vi "Main_FPGA old.vi"() -> ()   [LabVIEW 2018]
uses:
  <vilib>/rvi/eio/common/nirviEmuTemplateMethod_errors.vi
  <vilib>/rvi/Emulation/niFpgaGetClockAttributes.vi
  <vilib>/rvi/Emulation/niFpgaSctlEmulationGetInTimedLoop.vi
  <vilib>/rvi/Emulation/niFpgaEmulationReportErrorSimple.vi
  <vilib>/rvi/Emulation/niFpgaProcessEmulError.vi
  <vilib>/rvi/Emulation/niFpgaCriticalErrorInLSC.vi
  <vilib>/eio/EIONode/EIONode.xnode
  <vilib>/addons/control/pid/fpga.llb/XNode/niFpgaPID.xnode
panel:
  out "Mod6/unitR":bool
  out "Mod6/unitL":bool
  in  "Speed Loop Rate":u32=1000
  out "Mod8/AI15":fxp<+/-,24,5>
  out "Mod8/AI5":fxp<+/-,24,5>
  out "Mod8/AI4":fxp<+/-,24,5>
  out "Speed_cmd":fxp<+/-,17,6>
  in  "FeedFw_Ena":bool
  in  "ACC_FeedFw":fxp<+/-,16,5>
  out "Acc_2":fxp<+/-,36,10>
  out "Acc_1":fxp<+/-,36,10>
  in  "E-Acc_2":T1={"Gain"=1.0, "OffSet"=0.0}
  in  "E-Acc_1":T1={"Gain"=1.0, "OffSet"=0.0}
  in  "Speed Control Soll (%)":fxp<+/-,16,5>
  in  "Parameter Speed Control":fxp<+/-,16,5>
  in  "PID gains":T2={"proportional gain (Kc)"=1.5, "integral gain (Kc*Ts/Ti)"=0.19921875, "derivative gain (Kc*Td/Ts)"=0.0}
  in  "output range":T3={"output high"=10.0, "output low"=0.0}
  in  "Regler Speed Control":bool
  in  "Ist Speed Control":fxp<+/-,16,5>
  in  "Count (mSec) Fahrhebel":u32=25
  out "Tick Count(mSec) Hydraulic Wave":u32
  out "Count Hydraulic  Wave":i64
  out "Mod6/Fuel Transmitter":bool
  out "Mod6/DI30":bool
  out "Tick Count(mSec) Hydraulic":u32
  out "Count Hydraulic":i64
  in  "Mod7/Hydraulic clutch Set point":fxp<+/-,20,5>
  in  "Mod7/Hydraulic pump actuator Soll":fxp<+/-,20,5>
  in  "Mod7/Out 2":fxp<+/-,20,5>
  in  "Mod7/Out 1":fxp<+/-,20,5>
  out "DM Count":i64
  out "Tick Count(mSec)":u32
  in  "Mod4/DO30":bool
  in  "Mod4/Release Brake M":bool
  in  "Mod4/Richtung Engine Speed M":bool
  in  "Mod4/Release Engine Speed M":bool
  in  "Mod4/Richtung Up M":bool
  in  "Mod4/Release Up M":bool
  out "Mod6/End Position DOWN M":bool
  out "Mod6/DOWN M":bool
  out "Mod6/UP M":bool
  out "Mod6/End Position UP M":bool
  in  "Mod7/Up M Set point":fxp<+/-,20,5>
  in  "Mod7/Torque M Set point":fxp<+/-,20,5>
  out "Mod8/Engine Speed M":fxp<+/-,24,5>
  out "Mod8/Up M":fxp<+/-,24,5>
  in  "Mod4/Clutch":bool
  in  "Mod4/Temperature Control Release":bool
  in  "Mod4/Temperature Control OFF":bool
  in  "Mod4/Calibration ON Brake H":bool
  in  "Mod4/Unit ON Brake H":bool
  in  "Mod4/Brake Performance ON Brake H":bool
  in  "Mod4/Oil ON":bool
  in  "Mod3/Calibration Brake R":bool
  in  "Mod3/Unit ON Brake R":bool
  in  "Mod3/Brake Performance ON Brake R":bool
  in  "Mod3/Horn":bool
  in  "Mod3/DO20":bool
  in  "Mod3/Speed Control Release":bool
  in  "Mod3/DO18":bool
  in  "Mod3/Flashing light":bool
  in  "Mod3/Calibration ON Brake L":bool
  in  "Mod3/Unit ON Brake L":bool
  in  "Mod3/Brake Performance ON Brake L":bool
  in  "Mod3/Converter Clutch ON":bool
  in  "Mod3/Fuel Pump ON":bool
  in  "Mod3/Engine Ignition ON":bool
  in  "Mod3/Start Engine":bool
  in  "Mod3/Engine Pre Glow ON":bool
  in  "Cooling  Set point (°C)":fxp<+/-,16,5>
  in  "Heater Set point (°C)":fxp<+/-,16,5>
  in  "Alarm 24 ON":bool
  in  "Alarm 23 ON":bool
  in  "Alarm 22 ON":bool
  in  "Alarm 21 ON":bool
  in  "Alarm 20 ON":bool
  in  "Alarm 19 ON":bool
  in  "Alarm 18 ON":bool
  in  "Alarm 17 ON":bool
  in  "Alarm 16 ON":bool
  in  "Alarm 15 ON":bool
  in  "Alarm 14 ON":bool
  in  "Alarm 13 ON":bool
  in  "Alarm 12 ON":bool
  in  "Alarm 11 ON":bool
  in  "Alarm 10 ON":bool
  in  "Alarm 9 ON":bool
  in  "Alarm 8 ON":bool
  in  "Alarm 7 ON":bool
  in  "Alarm 6 ON":bool
  in  "Alarm 5 ON":bool
  in  "Alarm 4 ON":bool
  in  "Alarm 3 ON":bool
  out "Alarm":bool
  in  "Alarm 2 ON":bool
  in  "Alarm 1 ON":bool
  in  "Alarm ON":bool
  in  "STOP":bool
  out "Mod8/Kal 2 Brake H":fxp<+/-,24,5>
  out "Mod8/Kal 1 Brake H":fxp<+/-,24,5>
  out "Mod8/Kal 2 Brake R":fxp<+/-,24,5>
  out "Mod8/Kal 1 Brake R":fxp<+/-,24,5>
  out "Mod8/Kal 2 Brake L":fxp<+/-,24,5>
  out "Mod8/Kal 1 Brake L":fxp<+/-,24,5>
  out "Mod8/Engine Speed Wave Sensor":fxp<+/-,24,5>
  out "Mod8/Speed Control":fxp<+/-,24,5>
  in  "Mod3/System Reset/ON":bool
  out "Mod6/Clutch open":bool
  out "Mod6/Clutch closed":bool
  out "Mod6/Alarm 25 Basement":bool
  out "Mod6/Unit L-R":bool
  out "Mod6/Unit H":bool
  out "Mod6/Unit H-L-R":bool
  out "Mod6/Sytem Ready":bool
  out "Mod6/Watchdog Ready":bool
  out "Mod6/Alarm 2 Brake back":bool
  out "Mod6/Alarm 1 Brake back":bool
  out "Mod6/Temperature Brake back":bool
  out "Mod6/Ready Brake back":bool
  out "Mod6/Error Brake back":bool
  out "Mod6/Alarm 24 Overload Warning Oil Heating":bool
  out "Mod6/Alarm 23 Overload Warning Oil Pump":bool
  out "Mod6/Alarm 22 max Oil Pressure":bool
  out "Mod6/Alarm 21 min Oil Pressure":bool
  out "Mod6/Alarm 20 max Oil Temperature":bool
  out "Mod6/Alarm 18 Oil Level":bool
  out "Mod6/Alarm 19 min Oil Pressure":bool
  out "Mod6/Alarm 17 Oil Pressure Difference":bool
  out "Mod5/Alarm 2 Brake R":bool
  out "Mod5/Alarm 1 Brake R":bool
  out "Mod5/Temperature Brake R":bool
  out "Mod5/Ready Brake R":bool
  out "Mod5/Error Brake R":bool
  out "Mod5/Alarm 16 Fundament 4":bool
  out "Mod5/Alarm 15 Fundament 3":bool
  out "Mod5/Alarm 14 Fundament 2":bool
  out "Mod5/Alarm 13 Fundament 1":bool
  out "Mod5/Alarm 12 Spring Element":bool
  out "Mod5/Alarm 11 Watchdog":bool
  out "Mod5/Alarm 10 Fuel Depot":bool
  out "Mod5/Alarm 9 IGBT_ON":bool
  out "Mod5/Alarm 2 Brake L":bool
  out "Mod5/Alarm 1 Brake L":bool
  out "Mod5/Temperature Brake L":bool
  out "Mod5/Ready Brake L":bool
  out "Mod5/Error Brake L":bool
  out "Mod5/Alarm 8 Cooling Water":bool
  out "Mod5/Alarm 7 Exhaust":bool
  out "Mod5/Alarm 6 CO2":bool
  out "Mod5/Alarm 5 Clutch":bool
  out "Mod5/Alarm 4 Speed Control":bool
  out "Mod5/Alarm 3 Flow Control Unit":bool
  out "Mod5/Alarm 2 Gas":bool
  out "Mod5/Alarm 1 Fire":bool
  out "Mod2/Engine Speed  H":fxp<+/-,20,5>
  out "Mod2/Engine Speed R":fxp<+/-,20,5>
  out "Mod2/Engine Speed  L":fxp<+/-,20,5>
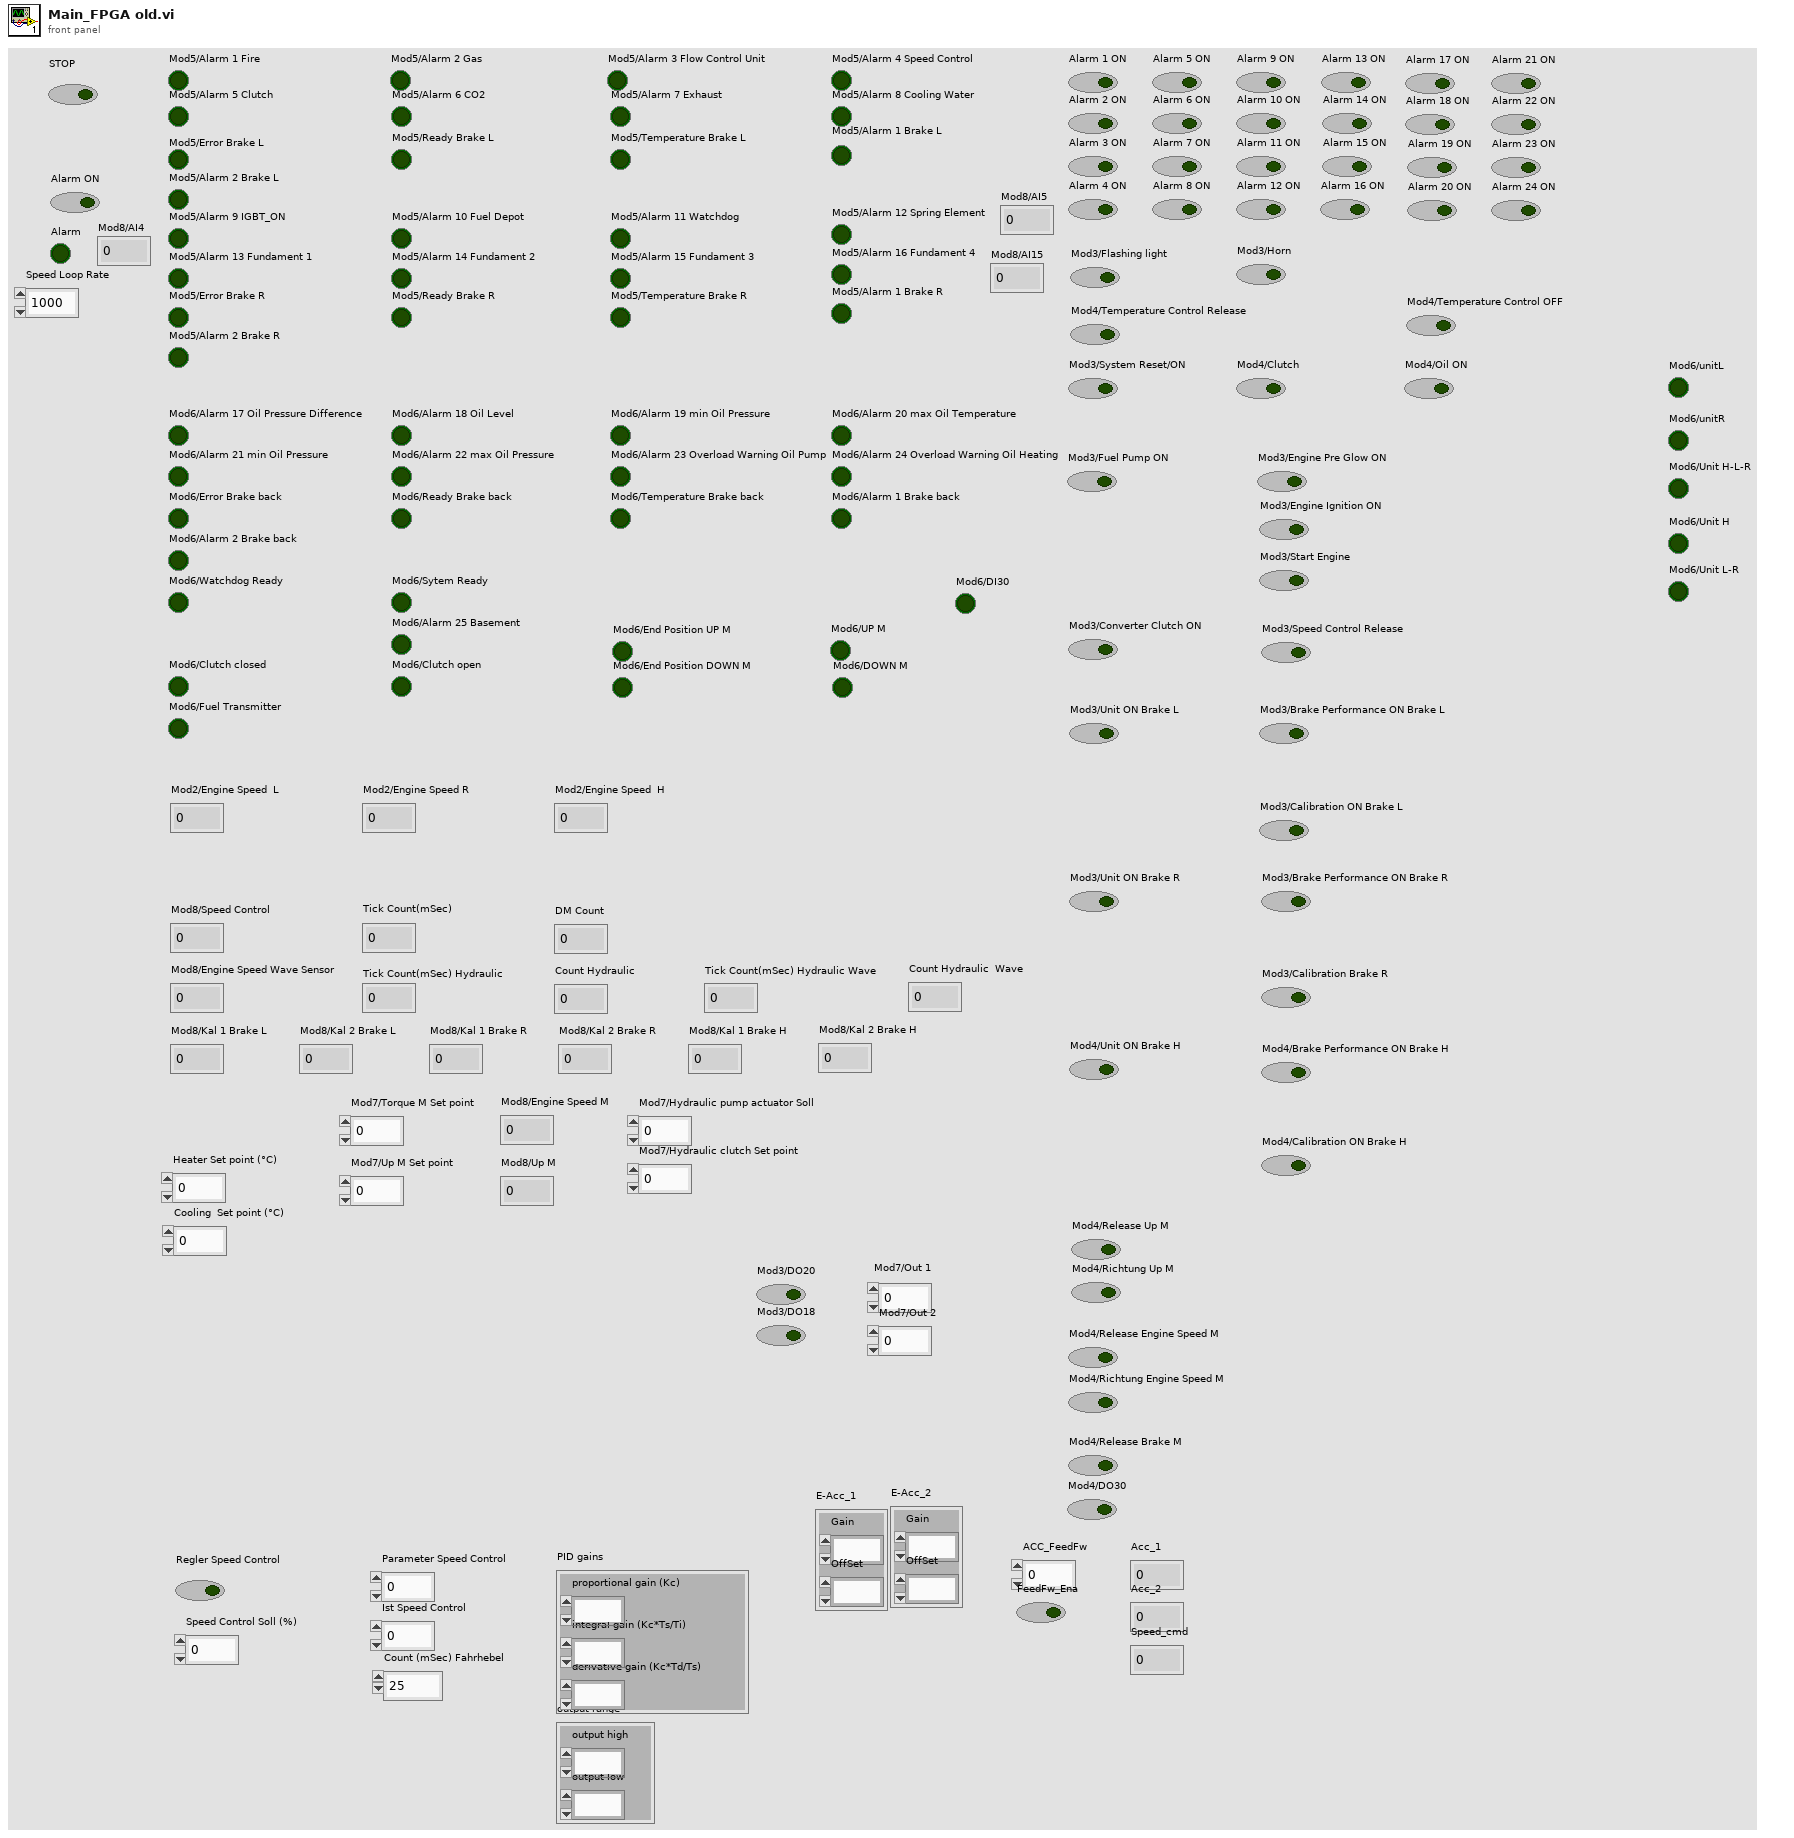
[diagram p1: front panel]
types:
  T1 = cluster{"Gain":fxp<+/-,20,5>, "OffSet":fxp<+/-,20,5>}
  T2 = cluster{"proportional gain (Kc)":fxp<+/-,16,8>, "integral gain (Kc*Ts/Ti)":fxp<+/-,16,8>, "derivative gain (Kc*Td/Ts)":fxp<+/-,16,8>}
  T3 = cluster{"output high":fxp<+/-,16,5>, "output low":fxp<+/-,16,5>}
  T4 = cluster{"proportional gain (Kc)":i16, "integral gain (Kc*Ts/Ti)":i16, "derivative gain (Kc*Td/Ts)":i16}
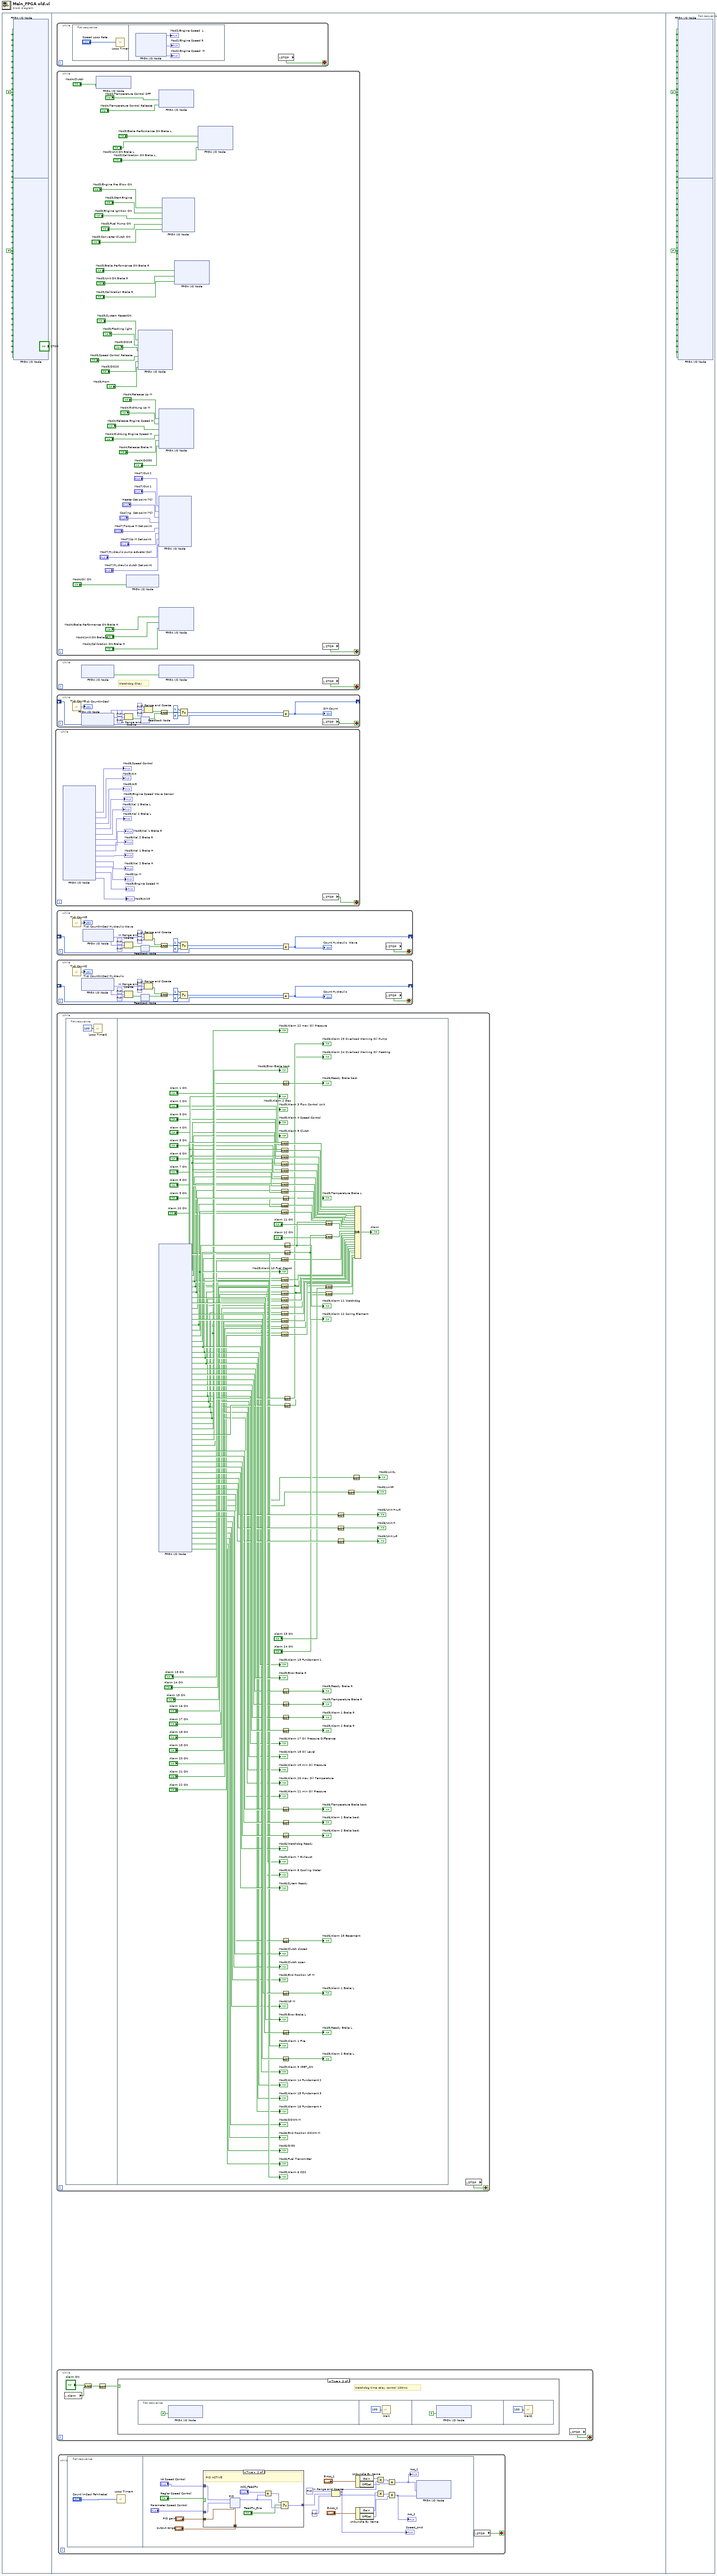
[diagram p0: block diagram]
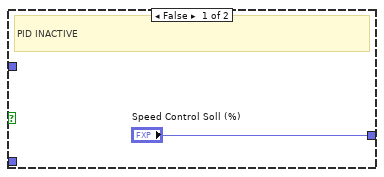
[diagram p2: hidden frame]
diagram:
  n1 = flat-sequence {
    frame #0 {
      w1 = FALSE ("Mod4/DO0")
      w2 = FALSE ("Mod3/DO0")
      n2 = xnode "FPGA I/O Node"("Mod4/DO0"=w1, "Mod4/DO1"=w1, "Mod4/DO2"=w1, "Mod4/DO3"=w1, "Mod4/DO4"=w1, "Mod4/DO5"=w1, "Mod4/DO6"=w1, "Mod4/DO7"=w1, "Mod4/DO8"=w1, "Mod4/DO9"=w1, "Mod4/DO10"=w1, "Mod4/DO11"=w1, "Mod4/DO12"=w1, "Mod4/DO13"=w1, "Mod4/DO14"=w1, "Mod4/DO15"=w1, "Mod4/DO16"=w1, "Mod4/DO17"=w1, "Mod4/DO18"=w1, "Mod4/DO19"=w1, "Mod4/DO20"=w1, "Mod4/DO21"=w1, "Mod4/DO22"=w1, "Mod4/DO23"=w1, "Mod4/DO24"=w1, "Mod4/DO25"=w1, "Mod4/DO26"=w1, "Mod4/DO27"=w1, "Mod4/DO28"=w1, "Mod4/DO29"=w1, "Mod4/DO30"=w1, "Mod4/DO31"=w1) -> ()  [unwired: 32 in, 32 out]
      n3 = xnode "FPGA I/O Node"("Mod3/DO0"=w2, "Mod3/DO1"=w2, "Mod3/DO2"=w2, "Mod3/DO3"=w2, "Mod3/DO4"=w2, "Mod3/DO5"=w2, "Mod3/DO6"=w2, "Mod3/DO7"=w2, "Mod3/DO8"=w2, "Mod3/DO9"=w2, "Mod3/DO10"=w2, "Mod3/DO11"=w2, "Mod3/DO12"=w2, "Mod3/DO13"=w2, "Mod3/DO14"=w2, "Mod3/DO15"=w2, "Mod3/DO16"=w2, "Mod3/DO17"=w2, "Mod3/DO18"=w2, "Mod3/DO19"=w2, "Mod3/DO20"=w2, "Mod3/DO21"=w2, "Mod3/DO22"=w2, "Mod3/DO23"=w2, "Mod3/DO24"=w2, "Mod3/DO25"=w2, "Mod3/DO26"=w2, "Mod3/DO27"=w2, "Mod3/DO28"=w2, "Mod3/DO29"=w2, "Mod3/DO30"=w2, "Mod3/DO31"=w2) -> ()  [unwired: 32 in, 32 out]
    }
    frame #1 {
      n4 = while {
        stop <- w6 stop-if-true
        n5 = xnode "FPGA I/O Node"() -> ("Mod8/AI3"=→"Mod8/Speed Control":fxp<+/-,24,5>, "Mod8/AI4"=→"Mod8/AI4":fxp<+/-,24,5>, "Mod8/AI5"=→"Mod8/AI5":fxp<+/-,24,5>, "Mod8/AI6"=→"Mod8/Engine Speed Wave Sensor":fxp<+/-,24,5>, "Mod8/AI7"=→"Mod8/Kal 1 Brake L":fxp<+/-,24,5>, "Mod8/AI8"=→"Mod8/Kal 2 Brake L":fxp<+/-,24,5>, "Mod8/AI9"=→"Mod8/Kal 1 Brake R":fxp<+/-,24,5>, "Mod8/AI10"=→"Mod8/Kal 2 Brake R":fxp<+/-,24,5>, "Mod8/AI11"=→"Mod8/Kal 1 Brake H":fxp<+/-,24,5>, "Mod8/AI12"=→"Mod8/Kal 2 Brake H":fxp<+/-,24,5>, "Mod8/AI13"=→"Mod8/Up M":fxp<+/-,24,5>, "Mod8/AI14"=→"Mod8/Engine Speed M":fxp<+/-,24,5>, "Mod8/AI15"=→"Mod8/AI15":fxp<+/-,24,5>)  [unwired: 16 in, 19 out]
        n6 = local read "STOP"() -> (w6:bool)
      }
      n7 = while {
        stop <- w17 stop-if-true
        n8 = flat-sequence {
          frame #0 {
            n9 = call "Loop Timer"("Count(uSec)"="Speed Loop Rate") -> ()  [unwired: 1 out]
          }
          frame #1 {
            n10 = xnode "FPGA I/O Node"() -> ("Mod2/AI0"=→"Mod2/Engine Speed  L":fxp<+/-,20,5>, "Mod2/AI1"=→"Mod2/Engine Speed R":fxp<+/-,20,5>, "Mod2/AI2"=→"Mod2/Engine Speed  H":fxp<+/-,20,5>)  [unwired: 3 in, 3 out]
          }
        }
        n11 = local read "STOP"() -> (w17:bool)
      }
      n12 = while {
        stop <- w167 stop-if-true
        n13 = xnode "FPGA I/O Node"("Mod4/DO24"="Mod4/Clutch") -> ()  [unwired: 1 in, 1 out]
        n14 = xnode "FPGA I/O Node"("Mod4/DO5"="Mod4/Oil ON") -> ()  [unwired: 1 in, 1 out]
        n15 = xnode "FPGA I/O Node"("Mod3/DO16"="Mod3/System Reset/ON", "Mod3/DO17"="Mod3/Flashing light", "Mod3/DO18"="Mod3/DO18", "Mod3/DO19"="Mod3/Speed Control Release", "Mod3/DO20"="Mod3/DO20", "Mod3/DO21"="Mod3/Horn") -> ()  [unwired: 6 in, 6 out]
        n16 = xnode "FPGA I/O Node"("Mod4/DO18"="Mod4/Temperature Control OFF", "Mod4/DO19"="Mod4/Temperature Control Release") -> ()  [unwired: 2 in, 2 out]
        n17 = xnode "FPGA I/O Node"("Mod4/DO25"="Mod4/Release Up M", "Mod4/DO26"="Mod4/Richtung Up M", "Mod4/DO27"="Mod4/Release Engine Speed M", "Mod4/DO28"="Mod4/Richtung Engine Speed M", "Mod4/DO29"="Mod4/Release Brake M", "Mod4/DO30"="Mod4/DO30") -> ()  [unwired: 6 in, 6 out]
        n18 = xnode "FPGA I/O Node"("Mod7/AO2"="Mod7/Out 2", "Mod7/AO1"="Mod7/Out 1", "Mod7/AO3"="Heater Set point (°C)", "Mod7/AO4"="Cooling  Set point (°C)", "Mod7/AO5"="Mod7/Torque M Set point", "Mod7/AO6"="Mod7/Up M Set point", "Mod7/AO7"="Mod7/Hydraulic pump actuator Soll", "Mod7/AO8"="Mod7/Hydraulic clutch Set point") -> ()  [unwired: 8 in, 8 out]
        n19 = xnode "FPGA I/O Node"("Mod4/DO10"="Mod4/Brake Performance ON Brake H", "Mod4/DO11"="Mod4/Unit ON Brake H", "Mod4/DO12"="Mod4/Calibration ON Brake H") -> ()  [unwired: 3 in, 3 out]
        n20 = xnode "FPGA I/O Node"("Mod3/DO0"="Mod3/Engine Pre Glow ON", "Mod3/DO1"="Mod3/Start Engine", "Mod3/DO2"="Mod3/Engine Ignition ON", "Mod3/DO3"="Mod3/Fuel Pump ON", "Mod3/DO4"="Mod3/Converter Clutch ON") -> ()  [unwired: 5 in, 5 out]
        n21 = xnode "FPGA I/O Node"("Mod3/DO26"="Mod3/Brake Performance ON Brake R", "Mod3/DO27"="Mod3/Unit ON Brake R", "Mod3/DO28"="Mod3/Calibration Brake R") -> ()  [unwired: 3 in, 3 out]
        n22 = xnode "FPGA I/O Node"("Mod3/DO10"="Mod3/Brake Performance ON Brake L", "Mod3/DO11"="Mod3/Unit ON Brake L", "Mod3/DO12"="Mod3/Calibration ON Brake L") -> ()  [unwired: 3 in, 3 out]
        n23 = local read "STOP"() -> (w167:bool)
      }
      n24 = while {
        stop <- w177 stop-if-true
        # "Watchdog Okay"
        n25 = xnode "FPGA I/O Node"() -> ("Mod6/DI16"=w178:bool)  [unwired: 1 in, 1 out]
        n26 = xnode "FPGA I/O Node"("Mod4/DO17"=w178) -> ()  [unwired: 1 in, 1 out]
        n27 = local read "STOP"() -> (w177:bool)
      }
      n28 = while {
        shift-right: [w121] -> _
        shift-left: _ -> [w122]
        stop <- w119 stop-if-true
        n29 = call "Tick Count"() -> ("Tick Count(mSec)"=→"Tick Count(mSec)":u32)
        n30 = xnode "FPGA I/O Node"() -> ("Mod8/AI14"=w116:fxp<+/-,24,5>)  [unwired: 1 in, 1 out]
        n31 = In Range and Coerce(upper limit=fxp<+/-,24,5> 3.0, x=w116, lower limit=fxp<+/-,24,5> 0.0) -> (In Range?=w117:bool)  [unwired: 1 out]
        n32 = feedback-in #1(w117) -> ()
        n33 = feedback #1() -> (w118:bool)  [unwired: 1 in]
        n34 = In Range and Coerce(upper limit=fxp<+/-,24,5> 6.0, x=w116, lower limit=fxp<+/-,24,5> 3.0) -> (In Range?=w113:bool)  [unwired: 1 out]
        n35 = And(x=w113, y=w118) -> (x .and. y?=w126:bool)
        n36 = Select(t=i64 1, s=w126, f=i64 0) -> (s? t:f=w123:i64)
        n37 = Add(x=w123, y=w122) -> (x+y=w121:i64)
        "DM Count" <- w121
        n38 = local read "STOP"() -> (w119:bool)
      }
      n39 = while {
        shift-right: [w89] -> _
        shift-left: _ -> [w90]
        stop <- w87 stop-if-true
        n40 = call "Tick Count3"() -> ("Tick Count(mSec)"=→"Tick Count(mSec) Hydraulic Wave":u32)
        n41 = xnode "FPGA I/O Node"() -> ("Mod2/AI3"=w84:fxp<+/-,20,5>)  [unwired: 1 in, 1 out]
        n42 = In Range and Coerce(upper limit=fxp<+/-,24,5> 3.0, x=w84, lower limit=fxp<+/-,24,5> 0.0) -> (In Range?=w85:bool)  [unwired: 1 out]
        n43 = feedback-in #2(w85) -> ()
        n44 = feedback #2() -> (w86:bool)  [unwired: 1 in]
        n45 = In Range and Coerce(upper limit=fxp<+/-,20,5> 6.0, x=w84, lower limit=fxp<+/-,20,5> 3.0) -> (In Range?=w81:bool)  [unwired: 1 out]
        n46 = And(x=w81, y=w86) -> (x .and. y?=w94:bool)
        n47 = Select(t=i64 1, s=w94, f=i64 0) -> (s? t:f=w91:i64)
        n48 = Add(x=w91, y=w90) -> (x+y=w89:i64)
        "Count Hydraulic  Wave" <- w89
        n49 = local read "STOP"() -> (w87:bool)
      }
      n50 = while {
        shift-right: [w105] -> _
        shift-left: _ -> [w106]
        stop <- w103 stop-if-true
        n51 = call "Tick Count2"() -> ("Tick Count(mSec)"=→"Tick Count(mSec) Hydraulic":u32)
        n52 = xnode "FPGA I/O Node"() -> ("Mod8/AI15"=w100:fxp<+/-,24,5>)  [unwired: 1 in, 1 out]
        n53 = In Range and Coerce(upper limit=fxp<+/-,24,5> 3.0, x=w100, lower limit=fxp<+/-,24,5> 0.0) -> (In Range?=w101:bool)  [unwired: 1 out]
        n54 = feedback-in #3(w101) -> ()
        n55 = feedback #3() -> (w102:bool)  [unwired: 1 in]
        n56 = In Range and Coerce(upper limit=fxp<+/-,24,5> 6.0, x=w100, lower limit=fxp<+/-,24,5> 3.0) -> (In Range?=w97:bool)  [unwired: 1 out]
        n57 = And(x=w97, y=w102) -> (x .and. y?=w110:bool)
        n58 = Select(t=i64 1, s=w110, f=i64 0) -> (s? t:f=w107:i64)
        n59 = Add(x=w107, y=w106) -> (x+y=w105:i64)
        "Count Hydraulic" <- w105
        n60 = local read "STOP"() -> (w103:bool)
      }
      n61 = while {
        stop <- w179 stop-if-true
        n62 = flat-sequence {
          frame #0 {
            n63 = call "Loop Timer2"("Count(mSec)"=u32 100) -> ()  [unwired: 1 out]
          }
          frame #1 {
            n64 = xnode "FPGA I/O Node"() -> ("Mod5/DI0"=w267:bool, "Mod5/DI1"=w265:bool, "Mod5/DI2"=w263:bool, "Mod5/DI3"=w256:bool, "Mod5/DI4"=w245:bool, "Mod5/DI5"=w246:bool, "Mod5/DI6"=w186:bool, "Mod5/DI7"=w187:bool, "Mod5/DI8"=→"Mod5/Error Brake L":bool, "Mod5/DI9"=w305:bool, "Mod5/DI10"=w304:bool, "Mod5/DI11"=w303:bool, "Mod5/DI12"=w302:bool, "Mod5/DI16"=w185:bool, "Mod5/DI17"=w242:bool, "Mod5/DI18"=w301:bool, "Mod5/DI19"=w300:bool, "Mod5/DI20"=w233:bool, "Mod5/DI21"=w230:bool, "Mod5/DI22"=w227:bool, "Mod5/DI23"=w224:bool, "Mod5/DI24"=→"Mod5/Error Brake R":bool, "Mod5/DI25"=w294:bool, "Mod5/DI26"=w298:bool, "Mod5/DI27"=w297:bool, "Mod5/DI28"=w296:bool, "Mod6/DI0"=w221:bool, "Mod6/DI1"=w218:bool, "Mod6/DI2"=w215:bool, "Mod6/DI3"=w212:bool, "Mod6/DI4"=w209:bool, "Mod6/DI5"=w206:bool, "Mod6/DI6"=w268:bool, "Mod6/DI7"=w295:bool, "Mod6/DI8"=→"Mod6/Error Brake back":bool, "Mod6/DI9"=w292:bool, "Mod6/DI10"=w291:bool, "Mod6/DI11"=w275:bool, "Mod6/DI12"=w290:bool, "Mod6/DI16"=→"Mod6/Watchdog Ready":bool, "Mod6/DI17"=→"Mod6/Sytem Ready":bool, "Mod6/DI18"=w287:bool, "Mod6/DI19"=w286:bool, "Mod6/DI20"=w285:bool, "Mod6/DI21"=w270:bool, "Mod6/DI22"=w184:bool, "Mod6/DI23"=w183:bool, "Mod6/DI24"=→"Mod6/Clutch closed":bool, "Mod6/DI25"=→"Mod6/Clutch open":bool, "Mod6/DI26"=→"Mod6/End Position UP M":bool, "Mod6/DI27"=→"Mod6/UP M":bool, "Mod6/DI28"=→"Mod6/DOWN M":bool, "Mod6/DI29"=→"Mod6/End Position DOWN M":bool, "Mod6/DI30"=→"Mod6/DI30":bool, "Mod6/DI31"=→"Mod6/Fuel Transmitter":bool)  [unwired: 55 in, 55 out]
            "Mod5/Alarm 1 Fire" <- w267
            "Mod5/Alarm 2 Gas" <- w265
            "Mod5/Alarm 3 Flow Control Unit" <- w263
            "Mod5/Alarm 4 Speed Control" <- w256
            "Mod5/Alarm 5 Clutch" <- w245
            "Mod5/Alarm 6 CO2" <- w246
            "Mod5/Alarm 7 Exhaust" <- w186
            "Mod5/Alarm 8 Cooling Water" <- w187
            "Mod5/Alarm 9 IGBT_ON" <- w185
            "Mod5/Alarm 10 Fuel Depot" <- w242
            "Mod5/Alarm 13 Fundament 1" <- w233
            "Mod5/Alarm 14 Fundament 2" <- w230
            "Mod5/Alarm 15 Fundament 3" <- w227
            "Mod5/Alarm 16 Fundament 4" <- w224
            "Mod6/Alarm 17 Oil Pressure Difference" <- w221
            "Mod6/Alarm 19 min Oil Pressure" <- w215
            "Mod6/Alarm 18 Oil Level" <- w218
            "Mod6/Alarm 20 max Oil Temperature" <- w212
            "Mod6/Alarm 21 min Oil Pressure" <- w209
            "Mod6/Alarm 22 max Oil Pressure" <- w206
            n65 = And(x=w267, y="Alarm 1 ON") -> (x .and. y?=w259:bool)
            n66 = And(x=w265, y="Alarm 2 ON") -> (x .and. y?=w260:bool)
            n67 = And(x=w263, y="Alarm 3 ON") -> (x .and. y?=w258:bool)
            n68 = And(x=w256, y="Alarm 4 ON") -> (x .and. y?=w257:bool)
            n69 = And(x=w245, y="Alarm 5 ON") -> (x .and. y?=w253:bool)
            n70 = And(x=w246, y="Alarm 6 ON") -> (x .and. y?=w252:bool)
            n71 = And(x=w186, y="Alarm 7 ON") -> (x .and. y?=w249:bool)
            n72 = And(x=w187, y="Alarm 8 ON") -> (x .and. y?=w247:bool)
            n73 = And(x=w185, y="Alarm 9 ON") -> (x .and. y?=w243:bool)
            n74 = And(x=w242, y="Alarm 10 ON") -> (x .and. y?=w240:bool)
            n75 = And(x=w233, y="Alarm 13 ON") -> (x .and. y?=w231:bool)
            n76 = And(x=w230, y="Alarm 14 ON") -> (x .and. y?=w229:bool)
            n77 = And(x=w227, y="Alarm 15 ON") -> (x .and. y?=w225:bool)
            n78 = And(x=w224, y="Alarm 16 ON") -> (x .and. y?=w223:bool)
            n79 = And(x=w221, y="Alarm 17 ON") -> (x .and. y?=w219:bool)
            n80 = And(x=w218, y="Alarm 18 ON") -> (x .and. y?=w216:bool)
            n81 = And(x=w215, y="Alarm 19 ON") -> (x .and. y?=w213:bool)
            n82 = And(x=w212, y="Alarm 20 ON") -> (x .and. y?=w210:bool)
            n83 = And(x=w209, y="Alarm 21 ON") -> (x .and. y?=w207:bool)
            n84 = And(x=w206, y="Alarm 22 ON") -> (x .and. y?=w204:bool)
            n85 = Not(x=w292) -> (.not. x?=→"Mod6/Ready Brake back":bool)
            n86 = Not(x=w304) -> (.not. x?=→"Mod5/Temperature Brake L":bool)
            n87 = Not(x=w294) -> (.not. x?=→"Mod5/Ready Brake R":bool)
            n88 = Not(x=w298) -> (.not. x?=→"Mod5/Temperature Brake R":bool)
            n89 = Not(x=w297) -> (.not. x?=→"Mod5/Alarm 1 Brake R":bool)
            n90 = Not(x=w296) -> (.not. x?=→"Mod5/Alarm 2 Brake R":bool)
            n91 = Not(x=w291) -> (.not. x?=→"Mod6/Temperature Brake back":bool)
            n92 = Not(x=w275) -> (.not. x?=→"Mod6/Alarm 1 Brake back":bool)
            n93 = Not(x=w290) -> (.not. x?=→"Mod6/Alarm 2 Brake back":bool)
            n94 = Not(x=w270) -> (.not. x?=→"Mod6/Alarm 25 Basement":bool)
            n95 = Not(x=w303) -> (.not. x?=→"Mod5/Alarm 1 Brake L":bool)
            n96 = Not(x=w305) -> (.not. x?=→"Mod5/Ready Brake L":bool)
            n97 = Not(x=w302) -> (.not. x?=→"Mod5/Alarm 2 Brake L":bool)
            n98 = Not(x=w301) -> (.not. x?=w239:bool)
            "Mod5/Alarm 11 Watchdog" <- w239
            n99 = Not(x=w300) -> (.not. x?=w236:bool)
            "Mod5/Alarm 12 Spring Element" <- w236
            n100 = Not(x=w268) -> (.not. x?=w203:bool)
            "Mod6/Alarm 23 Overload Warning Oil Pump" <- w203
            n101 = Not(x=w295) -> (.not. x?=w200:bool)
            "Mod6/Alarm 24 Overload Warning Oil Heating" <- w200
            n102 = And(x=w239, y="Alarm 11 ON") -> (x .and. y?=w237:bool)
            n103 = And(x=w236, y="Alarm 12 ON") -> (x .and. y?=w234:bool)
            n104 = And(x=w203, y="Alarm 23 ON") -> (x .and. y?=w201:bool)
            n105 = And(x=w200, y="Alarm 24 ON") -> (x .and. y?=w198:bool)
            n106 = Not(x=w287) -> (.not. x?=→"Mod6/Unit H-L-R":bool)
            n107 = Not(x=w286) -> (.not. x?=→"Mod6/Unit H":bool)
            n108 = Not(x=w285) -> (.not. x?=→"Mod6/Unit L-R":bool)
            n109 = Not(x=w183) -> (.not. x?=→"Mod6/unitR":bool)
            n110 = Not(x=w184) -> (.not. x?=→"Mod6/unitL":bool)
            n111 = Compound Arithmetic op=OR(w259, w260, w258, w257, w253, w252, w249, w247, w243, w240, w237, w234, w231, w229, w225, w223, w219, w216, w213, w210, w207, w204, w201, w198) -> (→"Alarm":bool)
          }
        }
        n112 = local read "STOP"() -> (w179:bool)
      }
      n113 = while {
        stop <- w168 stop-if-true
        n114 = local read "Alarm"() -> (w171:bool)
        n115 = And(x="Alarm ON", y=w171) -> (x .and. y?=w170:bool)
        n116 = Not(x=w170) -> (.not. x?=w169:bool)
        n117 = case shown="True" w169 {
          frame False {
          }
          frame True {
            # "Watchdog time relay control 100ms"
            n118 = flat-sequence {
              frame #0 {
                n119 = xnode "FPGA I/O Node"("Mod4/DO16"=FALSE) -> ()  [unwired: 1 in, 1 out]
              }
              frame #1 {
                n120 = call "Wait"("Count(mSec)"=u32 100) -> ()  [unwired: 1 out]
              }
              frame #2 {
                n121 = xnode "FPGA I/O Node"("Mod4/DO16"=TRUE) -> ()  [unwired: 1 in, 1 out]
              }
              frame #3 {
                n122 = call "Wait2"("Count(mSec)"=u32 100) -> ()  [unwired: 1 out]
              }
            }
          }
        }
        n123 = local read "STOP"() -> (w168:bool)
      }
      n124 = while {
        stop <- w22 stop-if-true
        n125 = flat-sequence {
          frame #0 {
            n126 = call "Loop Timer4"("Count(mSec)"="Count (mSec) Fahrhebel") -> ()  [unwired: 1 out]
          }
          frame #1 {
            n127 = case shown="True" "Regler Speed Control" {
              tunnel: "Ist Speed Control" -> [_ w52]
              tunnel: "Parameter Speed Control" -> [_ w51]
              tunnel: "PID gains" -> [_ w50]
              tunnel: "output range" -> [_ w49]
              tunnel: ["Speed Control Soll (%)" w44] -> w24
              frame False {
                # "PID INACTIVE"
              }
              frame True {
                # "PID ACTIVE"
                n128 = xnode "PID"("process variable"=w52, "setpoint"=w51, "PID gains"=w50, "output range"=w49) -> ("output"=w46:fxp<+/-,16,5>)  [unwired: 1 in]
                n129 = Add(x="ACC_FeedFw", y=w46) -> (x+y=w47:fxp<+/-,17,6>)
                n130 = Select(t=w47, s="FeedFw_Ena", f=w46) -> (s? t:f=w44:fxp<+/-,17,6>)
              }
            }
            n131 = In Range and Coerce(upper limit=fxp<+/-,17,6> 10.0, x=w24, lower limit=fxp<+/-,17,6> 0.0) -> (coerced(x)=w28:fxp<+/-,17,6>)  [unwired: 1 out]
            "Speed_cmd" <- w28
            n132 = Unbundle By Name("E-Acc_1") -> ("Gain"=w37:fxp<+/-,20,5>, "OffSet"=w35:fxp<+/-,20,5>)
            n133 = Unbundle By Name("E-Acc_2") -> ("Gain"=w32:fxp<+/-,20,5>, "OffSet"=w31:fxp<+/-,20,5>)
            n134 = Multiply(x=w37, y=w28) -> (x*y=w36:fxp<+/-,37,11>)
            n135 = Multiply(x=w32, y=w28) -> (x*y=w33:fxp<+/-,37,11>)
            n136 = Add(x=w36, y=w35) -> (x+y=w34:fxp<+/-,37,11>)
            "Acc_1" <- w34
            n137 = Add(x=w33, y=w31) -> (x+y=w30:fxp<+/-,37,11>)
            "Acc_2" <- w30
            n138 = xnode "FPGA I/O Node"("Mod7/AO14"=w34, "Mod7/AO15"=w30) -> ()  [unwired: 2 in, 2 out]
          }
        }
        n139 = local read "STOP"() -> (w22:bool)
      }
    }
    frame #2 {
      w307 = FALSE ("Mod4/DO0")
      w308 = FALSE ("Mod3/DO0")
      n140 = xnode "FPGA I/O Node"("Mod4/DO0"=w307, "Mod4/DO1"=w307, "Mod4/DO2"=w307, "Mod4/DO3"=w307, "Mod4/DO4"=w307, "Mod4/DO5"=w307, "Mod4/DO6"=w307, "Mod4/DO7"=w307, "Mod4/DO8"=w307, "Mod4/DO9"=w307, "Mod4/DO10"=w307, "Mod4/DO11"=w307, "Mod4/DO12"=w307, "Mod4/DO13"=w307, "Mod4/DO14"=w307, "Mod4/DO15"=w307, "Mod4/DO16"=w307, "Mod4/DO17"=w307, "Mod4/DO18"=w307, "Mod4/DO19"=w307, "Mod4/DO20"=w307, "Mod4/DO21"=w307, "Mod4/DO22"=w307, "Mod4/DO23"=w307, "Mod4/DO24"=w307, "Mod4/DO25"=w307, "Mod4/DO26"=w307, "Mod4/DO27"=w307, "Mod4/DO28"=w307, "Mod4/DO29"=w307, "Mod4/DO30"=w307, "Mod4/DO31"=w307) -> ()  [unwired: 32 in, 32 out]
      n141 = xnode "FPGA I/O Node"("Mod3/DO0"=w308, "Mod3/DO1"=w308, "Mod3/DO2"=w308, "Mod3/DO3"=w308, "Mod3/DO4"=w308, "Mod3/DO5"=w308, "Mod3/DO6"=w308, "Mod3/DO7"=w308, "Mod3/DO8"=w308, "Mod3/DO9"=w308, "Mod3/DO10"=w308, "Mod3/DO11"=w308, "Mod3/DO12"=w308, "Mod3/DO13"=w308, "Mod3/DO14"=w308, "Mod3/DO15"=w308, "Mod3/DO16"=w308, "Mod3/DO17"=w308, "Mod3/DO18"=w308, "Mod3/DO19"=w308, "Mod3/DO20"=w308, "Mod3/DO21"=w308, "Mod3/DO22"=w308, "Mod3/DO23"=w308, "Mod3/DO24"=w308, "Mod3/DO25"=w308, "Mod3/DO26"=w308, "Mod3/DO27"=w308, "Mod3/DO28"=w308, "Mod3/DO29"=w308, "Mod3/DO30"=w308, "Mod3/DO31"=w308) -> ()  [unwired: 32 in, 32 out]
    }
  }
